vi "Increment.vi"(8 "error in (no error)":errorcluster, 9 "Timeout (-1)":dbl[unit], 11 "Object Ref.":refnum<class "CS++Reference.lvclass">) -> (0 "error out":errorcluster, 1 "timed out?":bool, 3 "Object Ref. out":refnum<class "CS++Reference.lvclass">)   [LabVIEW 2012, in "CS++Core-Examples.lvlib" / "Example.lvclass"]
doc: "Increment Number attribute."
uses:
  Example.lvclass
  Core/Classes/CS++BaseClasses/Reference/CS++Reference.lvclass
  Example.lvclass/Example.ctl
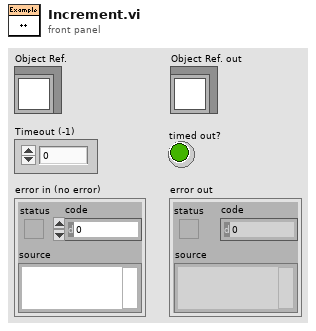
[diagram p1: front panel]
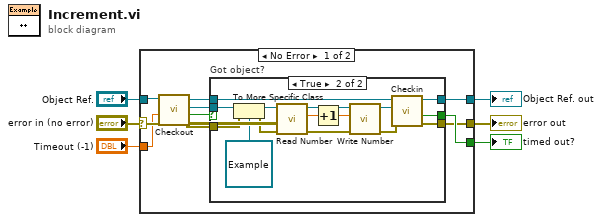
[diagram p0: block diagram]
diagram:
  n1 = case shown="No Error" "error in (no error)" {
    selector: "error in (no error)" -> [w8 w35]
    tunnel: [w9 w35] -> w5
    tunnel: [w11 w34] -> w3
    tunnel: "Object Ref." -> [w12 w34]
    tunnel: [w10 _] -> w2
    tunnel: "Timeout (-1)" -> [w7 _]
    frame No Error {
      n2 = call "Checkout.vi"("error in (no error)"=w8, "Timeout (-1)"=w7, "Object Reference"=w12) -> ("error out"=w15:errorcluster, "Object valid??"=w14:bool, "Object"=w16:refnum<class "CS++Base.lvclass">, "Object Reference out"=w13:refnum<class "CS++Reference.lvclass">)  [unwired: 5 in]
      n3 = case "Got object?" shown="True" w14 {
        tunnel: w16 -> [_ w33]
        tunnel: w15 -> [w17 w30]
        tunnel: w13 -> [w18 w28]
        tunnel: [w18 w27] -> w11
        tunnel: [w17 w26] -> w9
        tunnel: [_ w19] -> w10
        frame False {
        }
        frame True {
          n4 = To More Specific Class(target class=refnum<class "Example.lvclass"> refnum ("CS++Core-Examples.lvlib:Example.lvclass"), reference=w33, error in=w30) -> (specific class reference=w32:refnum<class "Example.lvclass">, error out=w29:errorcluster)
          n5 = call "Read Number.vi"("error in (no error)"=w29, "Example in"=w32) -> ("error out"=w23:errorcluster, "Number"=w25:dbl, "Example out"=w24:refnum<class "Example.lvclass">)  [unwired: 7 in]
          n6 = Increment(x=w25) -> (x+1=w22:dbl)
          n7 = call "Write Number.vi"("error in (no error)"=w23, "Number"=w22, "Example in"=w24) -> ("error out"=w20:errorcluster, "Example out"=w21:refnum<class "Example.lvclass">)  [unwired: 7 in]
          n8 = call "Checkin.vi"("error in (no error)"=w20, "Object"=w21, "Object Reference"=w28) -> ("error out"=w26:errorcluster, "timed out?"=w19:bool, "Object Reference out"=w27:refnum<class "CS++Reference.lvclass">)  [unwired: 6 in]
        }
      }
    }
    frame Error {
    }
  }
  "error out" <- w5
  "Object Ref. out" <- w3
  "timed out?" <- w2
